vi "initializeDefaultFont.vi"(8 "error in (no error)":errorcluster, 11 "Heading 2 in":refnum<class "Heading 2.lvclass">) -> (0 "error out":errorcluster, 3 "Heading 2 out":refnum<class "Heading 2.lvclass">)   [LabVIEW 2020, in "Styles.lvlib" / "Heading 2.lvclass"]
uses:
  Heading 2.lvclass
  Heading/Heading.lvclass
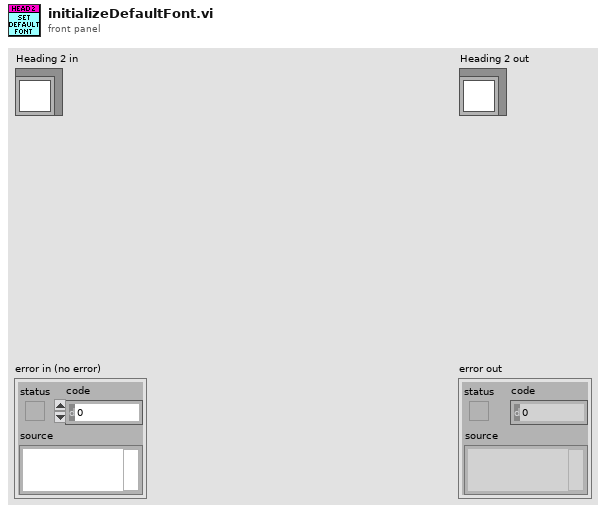
[diagram p1: front panel]
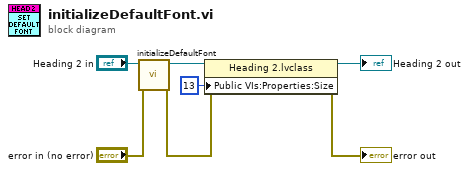
[diagram p0: block diagram]
diagram:
  n1 = call-parent "initializeDefaultFont.vi"("error in (no error)"="error in (no error)", "Heading in"="Heading 2 in") -> ("error out"=w2:errorcluster, "Heading out"=w7:refnum<class "Heading 2.lvclass">)  [unwired: 8 in]
  n2 = property class="Heading 2.lvclass"(reference=w7, error in=w2, "Public VIs:Properties:Size"=13 ("Style:Size")) -> (reference out=→"Heading 2 out":refnum<class "Heading 2.lvclass">, error out=→"error out":errorcluster)
